vi "modeMaintenance.vi"(11 "Array":string[](array[string])) -> (2 "advanceButton":i32, 3 "modeButton":i32)   [LabVIEW 2018]
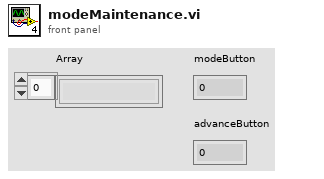
[diagram p1: front panel]
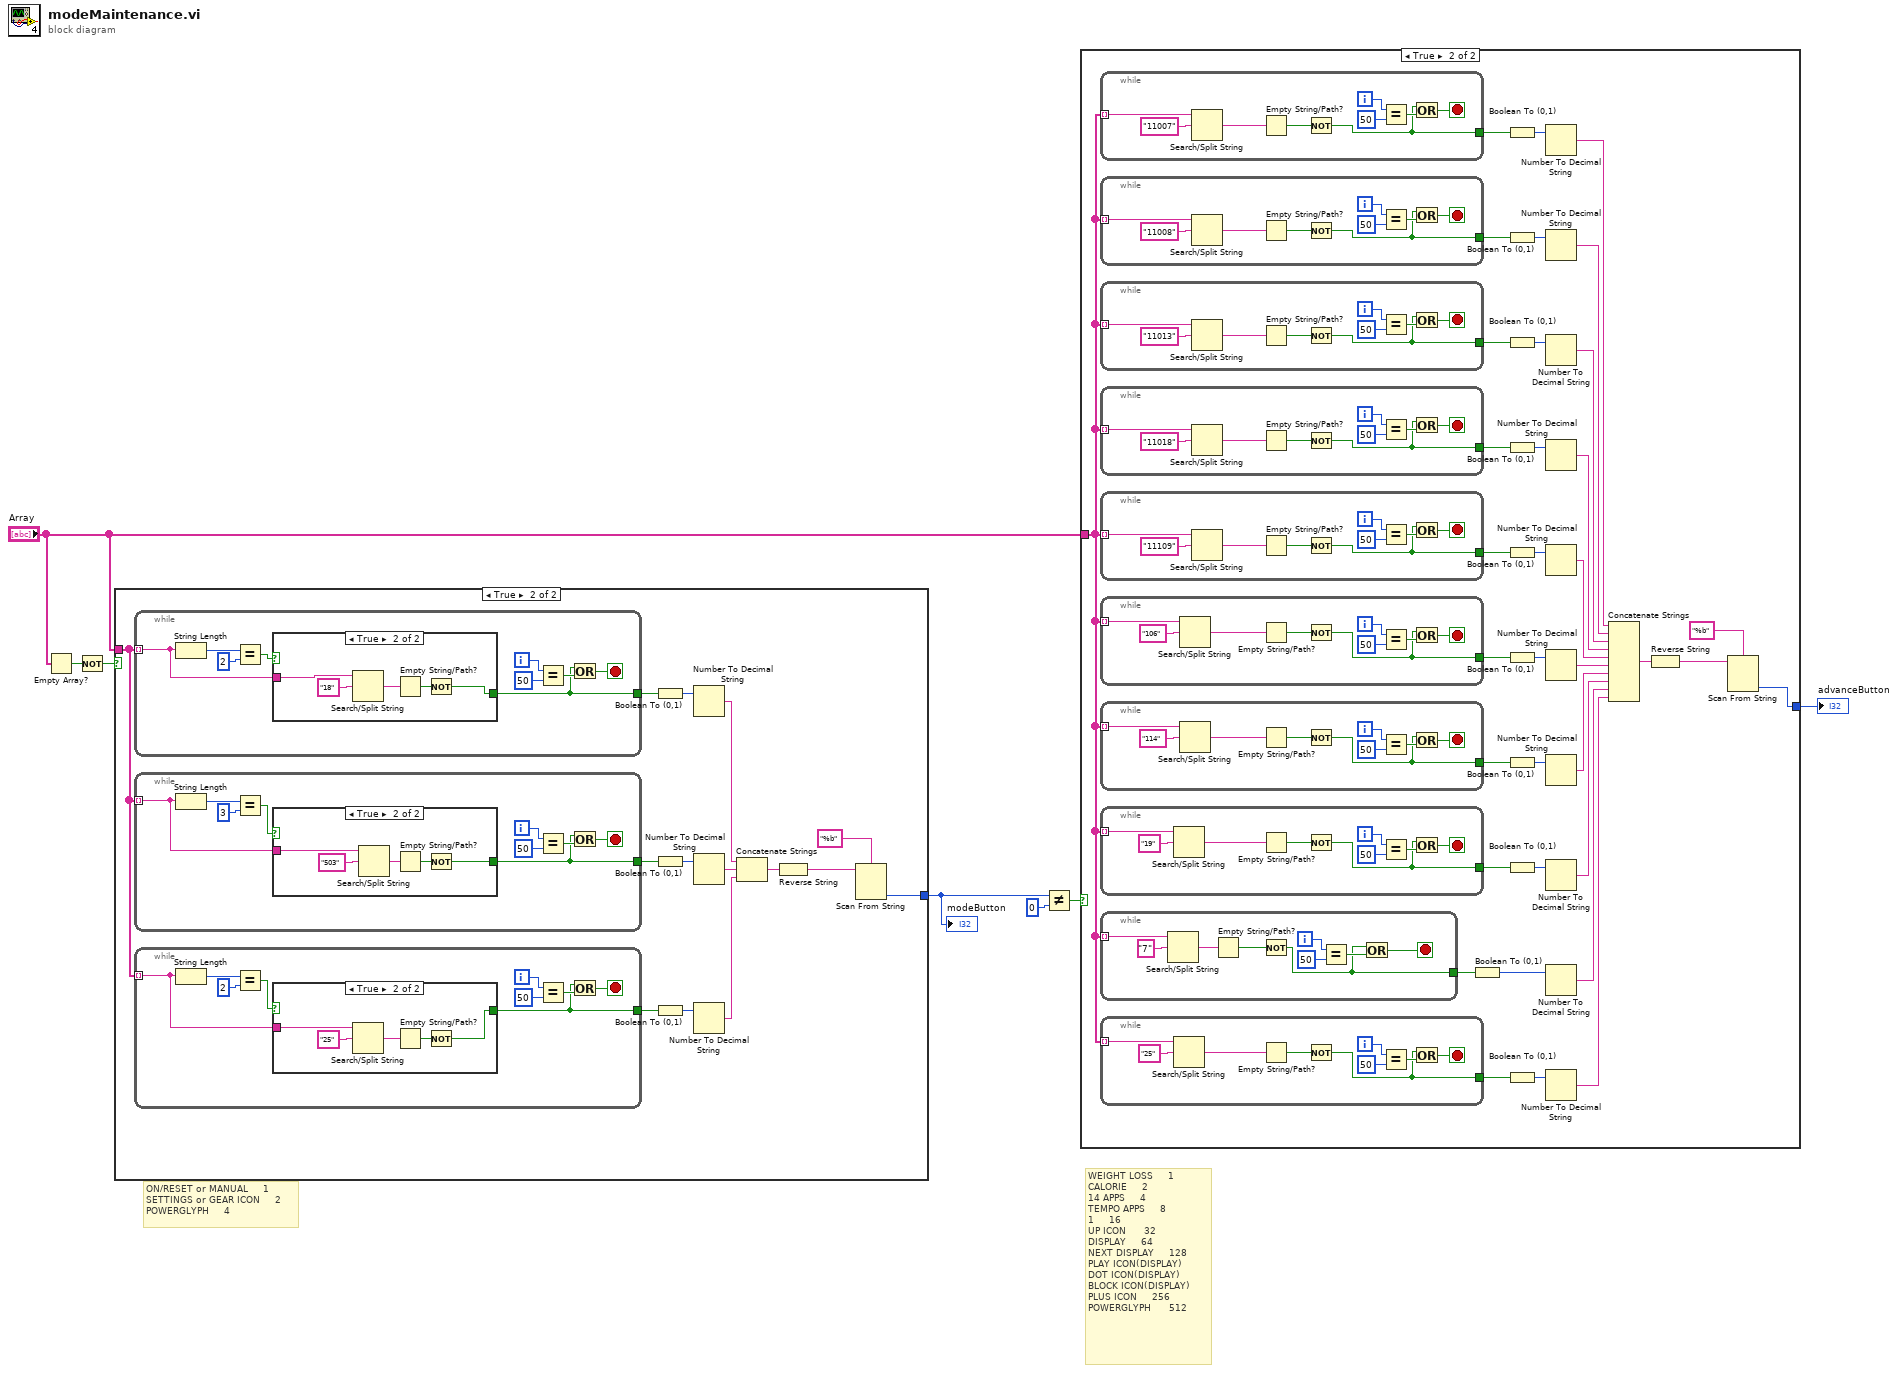
[diagram p0: block diagram]
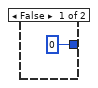
[diagram p2: hidden frame]
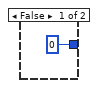
[diagram p3: hidden frame]
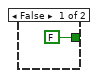
[diagram p4: hidden frame]
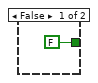
[diagram p5: hidden frame]
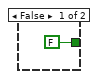
[diagram p6: hidden frame]
diagram:
  # "WEIGHT LOSS     1\nCALORIE     2\n14 APPS     4\nTEMPO APPS     8\n1     16\nUP ICON      32    \nDISPLAY     64\nNEXT DISPLAY     128\nPLAY ICON(DISPLAY)\nDOT ICON(DISPLAY)\nBLOCK ICON(DISPLAY)\nPLUS ICON     256\nPOWERGLYPH      512"
  # "ON/RESET or MANUAL     1\nSETTINGS or GEAR ICON     2\nPOWERGLYPH     4"
  n1 = Empty Array?(array="Array") -> (empty?=w3:bool)
  n2 = Not(x=w3) -> (.not. x?=w2:bool)
  n3 = case shown="True" w2 {
    tunnel: "Array" -> [_ w11]
    tunnel: [0 w14] -> w5
    frame False {
    }
    frame True {
      n4 = while {
        tunnel: w11 -> [w54] mode=indexing
        tunnel: [w53] -> w12
        i -> [w61]
        stop <- w59 stop-if-true
        n5 = String Length(string=w54) -> (length=w57:i32)
        n6 = Equal?(x=w57, y=2) -> (x = y?=w55:bool)
        n7 = case shown="True" w55 {
          tunnel: w54 -> [_ w64]
          tunnel: [FALSE w63] -> w53
          frame False {
          }
          frame True {
            n8 = Search/Split String(string=w64, search string/char (-)="18") -> (match + rest of string=w65:string)  [unwired: 1 in, 2 out]
            n9 = Empty String/Path?(string/path=w65) -> (empty?=w66:bool)
            n10 = Not(x=w66) -> (.not. x?=w63:bool)
          }
        }
        n11 = Equal?(x=w61, y=50) -> (x = y?=w58:bool)
        n12 = Or(x=w53, y=w58) -> (x .or. y?=w59:bool)
      }
      n13 = while {
        tunnel: w11 -> [w39] mode=indexing
        tunnel: [w38] -> w9
        i -> [w46]
        stop <- w44 stop-if-true
        n14 = String Length(string=w39) -> (length=w42:i32)
        n15 = Equal?(x=w42, y=3) -> (x = y?=w40:bool)
        n16 = case shown="True" w40 {
          tunnel: w39 -> [_ w49]
          tunnel: [FALSE w48] -> w38
          frame False {
          }
          frame True {
            n17 = Search/Split String(string=w49, search string/char (-)="503") -> (match + rest of string=w50:string)  [unwired: 1 in, 2 out]
            n18 = Empty String/Path?(string/path=w50) -> (empty?=w51:bool)
            n19 = Not(x=w51) -> (.not. x?=w48:bool)
          }
        }
        n20 = Equal?(x=w46, y=50) -> (x = y?=w43:bool)
        n21 = Or(x=w38, y=w43) -> (x .or. y?=w44:bool)
      }
      n22 = while {
        tunnel: w11 -> [w24] mode=indexing
        tunnel: [w23] -> w10
        i -> [w31]
        stop <- w29 stop-if-true
        n23 = String Length(string=w24) -> (length=w27:i32)
        n24 = Equal?(x=w27, y=2) -> (x = y?=w25:bool)
        n25 = case shown="True" w25 {
          tunnel: w24 -> [_ w34]
          tunnel: [FALSE w33] -> w23
          frame False {
          }
          frame True {
            n26 = Search/Split String(string=w34, search string/char (-)="25") -> (match + rest of string=w35:string)  [unwired: 1 in, 2 out]
            n27 = Empty String/Path?(string/path=w35) -> (empty?=w36:bool)
            n28 = Not(x=w36) -> (.not. x?=w33:bool)
          }
        }
        n29 = Equal?(x=w31, y=50) -> (x = y?=w28:bool)
        n30 = Or(x=w23, y=w28) -> (x .or. y?=w29:bool)
      }
      n31 = Boolean To (0,1)(Boolean=w12) -> (0, 1=w16:i16)
      n32 = Boolean To (0,1)(Boolean=w9) -> (0, 1=w17:i16)
      n33 = Boolean To (0,1)(Boolean=w10) -> (0, 1=w18:i16)
      n34 = Number To Decimal String(number=w16) -> (decimal integer string=w20:string)  [unwired: 1 in]
      n35 = Number To Decimal String(number=w17) -> (decimal integer string=w19:string)  [unwired: 1 in]
      n36 = Number To Decimal String(number=w18) -> (decimal integer string=w21:string)  [unwired: 1 in]
      n37 = Concatenate Strings(w20, w19, w21) -> (w22:string)
      n38 = Reverse String(1:w22) -> (0:w13:string)
      n39 = Scan From String(format string="%b", input string=w13) -> (output 1=w14:i32)  [unwired: 3 in, 3 out]
    }
  }
  "modeButton" <- w5
  n40 = Not Equal?(x=w5, y=0) -> (x != y?=w4:bool)
  n41 = case shown="True" w4 {
    tunnel: "Array" -> [_ w72]
    tunnel: [0 w70] -> w7
    frame False {
    }
    frame True {
      n42 = while {
        tunnel: w72 -> [w189] mode=indexing
        tunnel: [w185] -> w94
        i -> [w193]
        stop <- w191 stop-if-true
        n43 = Search/Split String(string=w189, search string/char (-)="11007") -> (match + rest of string=w186:string)  [unwired: 1 in, 2 out]
        n44 = Empty String/Path?(string/path=w186) -> (empty?=w187:bool)
        n45 = Not(x=w187) -> (.not. x?=w185:bool)
        n46 = Equal?(x=w193, y=50) -> (x = y?=w190:bool)
        n47 = Or(x=w185, y=w190) -> (x .or. y?=w191:bool)
      }
      n48 = while {
        tunnel: w72 -> [w180] mode=indexing
        tunnel: [w176] -> w95
        i -> [w184]
        stop <- w182 stop-if-true
        n49 = Search/Split String(string=w180, search string/char (-)="11008") -> (match + rest of string=w177:string)  [unwired: 1 in, 2 out]
        n50 = Empty String/Path?(string/path=w177) -> (empty?=w178:bool)
        n51 = Not(x=w178) -> (.not. x?=w176:bool)
        n52 = Equal?(x=w184, y=50) -> (x = y?=w181:bool)
        n53 = Or(x=w176, y=w181) -> (x .or. y?=w182:bool)
      }
      n54 = while {
        tunnel: w72 -> [w171] mode=indexing
        tunnel: [w167] -> w96
        i -> [w175]
        stop <- w173 stop-if-true
        n55 = Search/Split String(string=w171, search string/char (-)="11013") -> (match + rest of string=w168:string)  [unwired: 1 in, 2 out]
        n56 = Empty String/Path?(string/path=w168) -> (empty?=w169:bool)
        n57 = Not(x=w169) -> (.not. x?=w167:bool)
        n58 = Equal?(x=w175, y=50) -> (x = y?=w172:bool)
        n59 = Or(x=w167, y=w172) -> (x .or. y?=w173:bool)
      }
      n60 = while {
        tunnel: w72 -> [w153] mode=indexing
        tunnel: [w149] -> w92
        i -> [w157]
        stop <- w155 stop-if-true
        n61 = Search/Split String(string=w153, search string/char (-)="11018") -> (match + rest of string=w150:string)  [unwired: 1 in, 2 out]
        n62 = Empty String/Path?(string/path=w150) -> (empty?=w151:bool)
        n63 = Not(x=w151) -> (.not. x?=w149:bool)
        n64 = Equal?(x=w157, y=50) -> (x = y?=w154:bool)
        n65 = Or(x=w149, y=w154) -> (x .or. y?=w155:bool)
      }
      n66 = while {
        tunnel: w72 -> [w162] mode=indexing
        tunnel: [w158] -> w84
        i -> [w166]
        stop <- w164 stop-if-true
        n67 = Search/Split String(string=w162, search string/char (-)="11109") -> (match + rest of string=w159:string)  [unwired: 1 in, 2 out]
        n68 = Empty String/Path?(string/path=w159) -> (empty?=w160:bool)
        n69 = Not(x=w160) -> (.not. x?=w158:bool)
        n70 = Equal?(x=w166, y=50) -> (x = y?=w163:bool)
        n71 = Or(x=w158, y=w163) -> (x .or. y?=w164:bool)
      }
      n72 = while {
        tunnel: w72 -> [w126] mode=indexing
        tunnel: [w122] -> w80
        i -> [w130]
        stop <- w128 stop-if-true
        n73 = Search/Split String(string=w126, search string/char (-)="106") -> (match + rest of string=w123:string)  [unwired: 1 in, 2 out]
        n74 = Empty String/Path?(string/path=w123) -> (empty?=w124:bool)
        n75 = Not(x=w124) -> (.not. x?=w122:bool)
        n76 = Equal?(x=w130, y=50) -> (x = y?=w127:bool)
        n77 = Or(x=w122, y=w127) -> (x .or. y?=w128:bool)
      }
      n78 = while {
        tunnel: w72 -> [w117] mode=indexing
        tunnel: [w113] -> w74
        i -> [w121]
        stop <- w119 stop-if-true
        n79 = Search/Split String(string=w117, search string/char (-)="114") -> (match + rest of string=w114:string)  [unwired: 1 in, 2 out]
        n80 = Empty String/Path?(string/path=w114) -> (empty?=w115:bool)
        n81 = Not(x=w115) -> (.not. x?=w113:bool)
        n82 = Equal?(x=w121, y=50) -> (x = y?=w118:bool)
        n83 = Or(x=w113, y=w118) -> (x .or. y?=w119:bool)
      }
      n84 = while {
        tunnel: w72 -> [w108] mode=indexing
        tunnel: [w104] -> w73
        i -> [w112]
        stop <- w110 stop-if-true
        n85 = Search/Split String(string=w108, search string/char (-)="19") -> (match + rest of string=w105:string)  [unwired: 1 in, 2 out]
        n86 = Empty String/Path?(string/path=w105) -> (empty?=w106:bool)
        n87 = Not(x=w106) -> (.not. x?=w104:bool)
        n88 = Equal?(x=w112, y=50) -> (x = y?=w109:bool)
        n89 = Or(x=w104, y=w109) -> (x .or. y?=w110:bool)
      }
      n90 = while {
        tunnel: w72 -> [w144] mode=indexing
        tunnel: [w140] -> w85
        i -> [w148]
        stop <- w146 stop-if-true
        n91 = Search/Split String(string=w144, search string/char (-)="7") -> (match + rest of string=w141:string)  [unwired: 1 in, 2 out]
        n92 = Empty String/Path?(string/path=w141) -> (empty?=w142:bool)
        n93 = Not(x=w142) -> (.not. x?=w140:bool)
        n94 = Equal?(x=w148, y=50) -> (x = y?=w145:bool)
        n95 = Or(x=w140, y=w145) -> (x .or. y?=w146:bool)
      }
      n96 = while {
        tunnel: w72 -> [w135] mode=indexing
        tunnel: [w131] -> w86
        i -> [w139]
        stop <- w137 stop-if-true
        n97 = Search/Split String(string=w135, search string/char (-)="25") -> (match + rest of string=w132:string)  [unwired: 1 in, 2 out]
        n98 = Empty String/Path?(string/path=w132) -> (empty?=w133:bool)
        n99 = Not(x=w133) -> (.not. x?=w131:bool)
        n100 = Equal?(x=w139, y=50) -> (x = y?=w136:bool)
        n101 = Or(x=w131, y=w136) -> (x .or. y?=w137:bool)
      }
      n102 = Boolean To (0,1)(Boolean=w85) -> (0, 1=w90:i16)
      n103 = Boolean To (0,1)(Boolean=w94) -> (0, 1=w97:i16)
      n104 = Boolean To (0,1)(Boolean=w95) -> (0, 1=w98:i16)
      n105 = Boolean To (0,1)(Boolean=w96) -> (0, 1=w99:i16)
      n106 = Boolean To (0,1)(Boolean=w92) -> (0, 1=w93:i16)
      n107 = Boolean To (0,1)(Boolean=w84) -> (0, 1=w91:i16)
      n108 = Boolean To (0,1)(Boolean=w80) -> (0, 1=w83:i16)
      n109 = Boolean To (0,1)(Boolean=w74) -> (0, 1=w82:i16)
      n110 = Boolean To (0,1)(Boolean=w73) -> (0, 1=w81:i16)
      n111 = Boolean To (0,1)(Boolean=w86) -> (0, 1=w89:i16)
      n112 = Number To Decimal String(number=w97) -> (decimal integer string=w101:string)  [unwired: 1 in]
      n113 = Number To Decimal String(number=w98) -> (decimal integer string=w100:string)  [unwired: 1 in]
      n114 = Number To Decimal String(number=w99) -> (decimal integer string=w102:string)  [unwired: 1 in]
      n115 = Number To Decimal String(number=w93) -> (decimal integer string=w88:string)  [unwired: 1 in]
      n116 = Number To Decimal String(number=w91) -> (decimal integer string=w87:string)  [unwired: 1 in]
      n117 = Number To Decimal String(number=w83) -> (decimal integer string=w79:string)  [unwired: 1 in]
      n118 = Number To Decimal String(number=w82) -> (decimal integer string=w78:string)  [unwired: 1 in]
      n119 = Number To Decimal String(number=w81) -> (decimal integer string=w77:string)  [unwired: 1 in]
      n120 = Number To Decimal String(number=w90) -> (decimal integer string=w76:string)  [unwired: 1 in]
      n121 = Number To Decimal String(number=w89) -> (decimal integer string=w75:string)  [unwired: 1 in]
      n122 = Concatenate Strings(w101, w100, w102, w88, w87, w79, w78, w77, w76, w75) -> (w103:string)
      n123 = Reverse String(1:w103) -> (0:w69:string)
      n124 = Scan From String(format string="%b", input string=w69) -> (output 1=w70:i32)  [unwired: 3 in, 3 out]
    }
  }
  "advanceButton" <- w7
